vi "_emi_New Loop Numb.vi"(2 "Loop Enable (F)":bool, 7 "Loop Index":u16, 9 "error in (no error)":errorcluster) -> (6 "Loop ID":u16, 10 "error out":errorcluster)   [LabVIEW 2010]
doc: "Create a new loop, input loop index or enum (must be uniqe to the loop)"
uses:
  _emi_Loop control int action.ctl
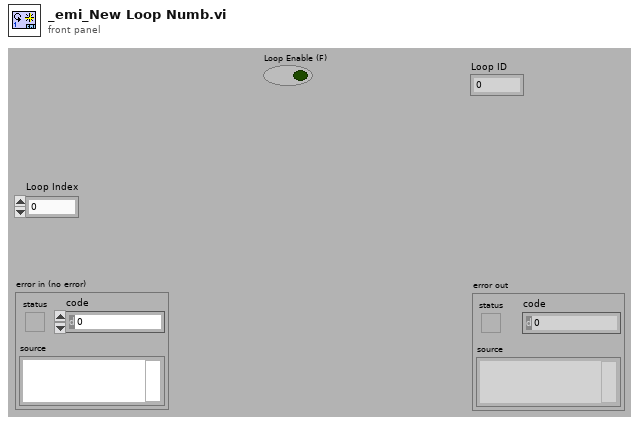
[diagram p1: front panel]
types:
  T1 = typedef "_emi_Loop control int action.ctl" = enum16{"Init index", "Get index", "Set index", "Get Size"}
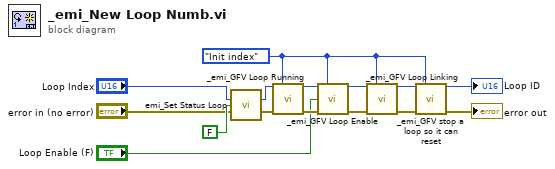
[diagram p0: block diagram]
diagram:
  w5 = _emi_Loop_control_int_action."Init index" ("Action(Get Index)")
  n1 = call "emi_Set Status Loop.vi"("Loop ID in"="Loop Index", "Running?"=FALSE, "error in (no error)"="error in (no error)") -> ("Loop ID out"=w9:u16, "error out"=w11:errorcluster)  [unwired: 11 in]
  n2 = call "_emi_GFV Loop Running.vi"("Loop Index/Numb"=w9, "Action(Get Index)"=w5, "error in (no error)"=w11) -> ("Index out"=w12:u16, "error out"=w10:errorcluster)  [unwired: 9 in, 2 out]
  n3 = call "_emi_GFV Loop Enable.vi"("Loop Index/Numb"=w12, "Action(Get Index)"=w5, "Loop enable In(T)"="Loop Enable (F)", "error in (no error)"=w10) -> ("Index out"=w3:u16, "error out"=w7:errorcluster)  [unwired: 8 in, 2 out]
  n4 = call "_emi_GFV Loop Linking.vi"("Loop Index/Numb"=w3, "Action(Get Index)"=w5, "error in (no error)"=w7) -> ("Index out"=w2:u16, "error out"=w6:errorcluster)  [unwired: 9 in, 2 out]
  n5 = call "_emi_GFV stop a loop so it can reset.vi"("Loop Index/Numb"=w2, "Action(Get Index)"=w5, "error in (no error)"=w6) -> ("Index out"=→"Loop ID":u16, "error out"=→"error out":errorcluster)  [unwired: 9 in, 2 out]
